vi "cam_dll_fgv.vi"(7 "cmd":enum16{"update", "grab", "ini", "close"}(ring), 8 "error in":errorcluster, 9 "nYposition":i32, 10 "nXposition":i32, 11 "IPadderss":string) -> (0 "error out":errorcluster, 3 "temp":dbl)   [LabVIEW 2013]
uses:
  <userlib>/test_win32dll_d/test_win32dll_d.lvlib
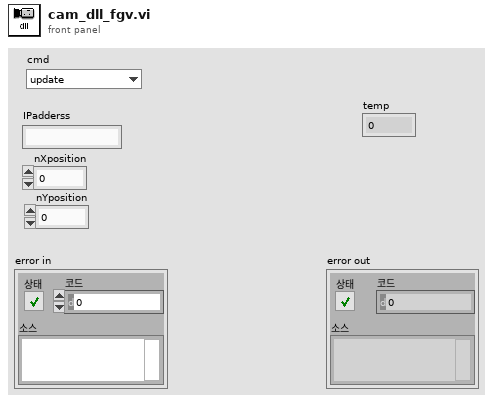
[diagram p1: front panel]
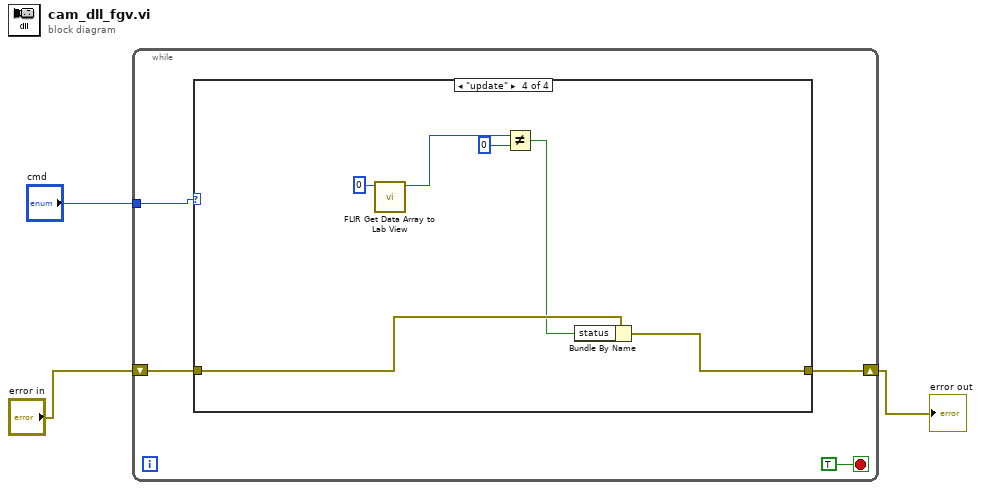
[diagram p0: block diagram]
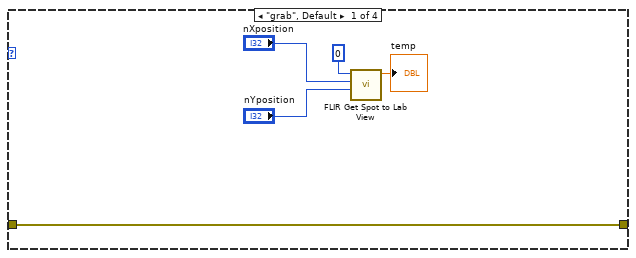
[diagram p2: hidden frame]
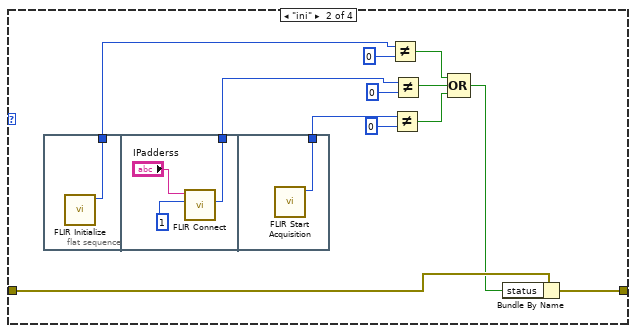
[diagram p3: hidden frame]
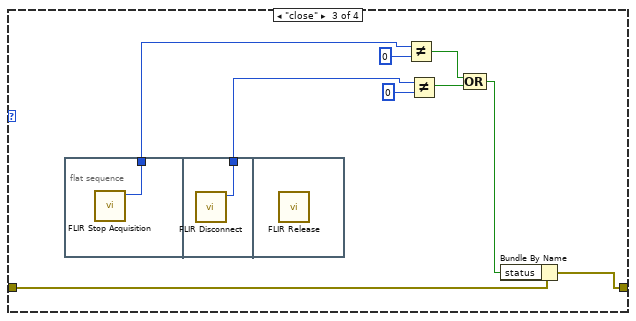
[diagram p4: hidden frame]
diagram:
  n1 = while {
    shift-right: [w4] -> w1
    shift-left: "error in" -> [w5]
    tunnel: "cmd" -> [w6]
    stop <- TRUE stop-if-true
    n2 = case shown="\"update\"" w6 {
      tunnel: w5 -> [w8 w17 w33 w43]
      tunnel: [w8 w15 w32 w41] -> w4
      frame "grab", Default {
        n3 = call <userlib>:"FLIR Get Spot to Lab View.vi"("nYposition"="nYposition", "nXposition"="nXposition", "nTemperatureType"=0) -> ("function return"=→"temp":dbl)  [unwired: 8 in]
      }
      frame "ini" {
        n4 = flat-sequence {
          tunnel: [w25] -> w23
          tunnel: [w26] -> w14
          tunnel: [w29] -> w13
          frame #0 {
            n5 = call <userlib>:"FLIR Initialize.vi"() -> ("function return"=w25:i32)  [unwired: 11 in]
          }
          frame #1 {
            n6 = call <userlib>:"FLIR Connect.vi"("nValue"=1, "IPadderss"="IPadderss") -> ("function return"=w26:i32)  [unwired: 8 in, 1 out]
          }
          frame #2 {
            n7 = call <userlib>:"FLIR Start Acquisition.vi"() -> ("function return"=w29:i32)  [unwired: 11 in]
          }
        }
        n8 = Not Equal?(x=w23, y=0) -> (x != y?=w18:bool)
        n9 = Not Equal?(x=w13, y=0) -> (x != y?=w20:bool)
        n10 = Not Equal?(x=w14, y=0) -> (x != y?=w19:bool)
        n11 = Compound Arithmetic op=OR(w18, w19, w20) -> (w16:bool)
        n12 = Bundle By Name(cluster=w17, "status"=w16) -> (w15:errorcluster)
      }
      frame "close" {
        n13 = flat-sequence {
          tunnel: [w39] -> w34
          tunnel: [w40] -> w30
          frame #0 {
            n14 = call <userlib>:"FLIR Stop Acquisition.vi"() -> ("function return"=w39:i32)  [unwired: 11 in]
          }
          frame #1 {
            n15 = call <userlib>:"FLIR Disconnect.vi"() -> ("function return"=w40:i32)  [unwired: 11 in]
          }
          frame #2 {
            n16 = call <userlib>:"FLIR Release.vi"() -> ()  [unwired: 12 in]
          }
        }
        n17 = Not Equal?(x=w34, y=0) -> (x != y?=w35:bool)
        n18 = Not Equal?(x=w30, y=0) -> (x != y?=w36:bool)
        n19 = Compound Arithmetic op=OR(w35, w36) -> (w31:bool)
        n20 = Bundle By Name(cluster=w33, "status"=w31) -> (w32:errorcluster)
      }
      frame "update" {
        n21 = call <userlib>:"FLIR Get Data Array to Lab View.vi"("nFormat"=0) -> ("function return"=w44:i32)  [unwired: 10 in]
        n22 = Not Equal?(x=w44, y=0) -> (x != y?=w42:bool)
        n23 = Bundle By Name(cluster=w43, "status"=w42) -> (w41:errorcluster)
      }
    }
  }
  "error out" <- w1
